vi "Codec_CMD_0_Will.vi"(8 "error in (no error)":errorcluster, 10 "CMD":u32, 11 "SecureMqttCodec in":refnum<class "SecureMqttCodec.lvclass">) -> (0 "error out":errorcluster, 2 "<JSON>":string, 3 "SecureMqttCodec out":refnum<class "SecureMqttCodec.lvclass">)   [LabVIEW 2020, in "SecureMqttCodec.lvclass"]
uses:
  SecureMqttCodec.lvclass
  SecureMqttCodec.lvclass/SecureMqttCodec.ctl
  <vilib>/LabVIEW Open Source Project/Epoch Date & Time/epoch.UNIX/Epoch.UNIX.lvclass
  C:/Program Files/National Instruments/LabVIEW 2020/vi.lib/LabVIEW Open Source Project/Epoch Date & Time/epoch/Epoch.lvclass
  <vilib>/addons/JSON API/JSON Scalar/JSON Scalar.lvclass
  C:/Program Files/National Instruments/LabVIEW 2020/vi.lib/addons/JSON API/JSON Value/JSON Value.lvclass
  <vilib>/LabVIEW Open Source Project/Epoch Date & Time/Get Epoch Time.vi
  <vilib>/addons/JSON API/JSON Scalar/Set I64.vi
  <vilib>/addons/JSON API/JSON Scalar/Set U32.vi
  <vilib>/addons/JSON API/JSON Scalar/Set String.vi
  <vilib>/addons/JSON API/JSON Value/Get as JSON string (pretty).vi
  <vilib>/addons/JSON API/JSON Value/JSON Value.lvclass
  <vilib>/addons/JSON API/Get Polymorphic/JSON GetSet.lvlib
panel:
  # "Command:\n0 -- Reg Client\n65535 -- Reg Will"
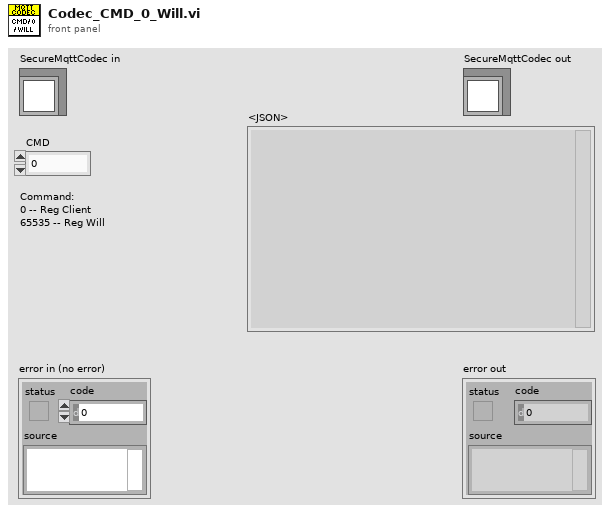
[diagram p1: front panel]
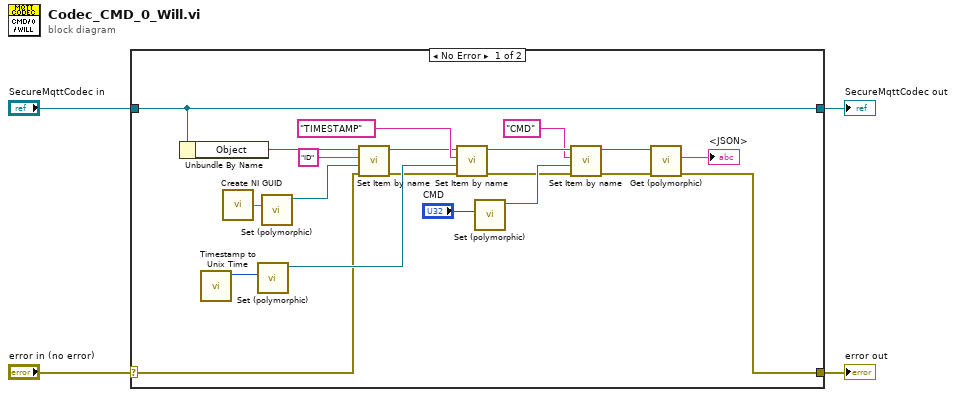
[diagram p0: block diagram]
diagram:
  n1 = case shown="No Error" "error in (no error)" {
    selector: "error in (no error)" -> [w9 w26]
    tunnel: [w6 w26] -> w3
    tunnel: [w24 w25] -> w1
    tunnel: "SecureMqttCodec in" -> [w24 w25]
    frame No Error {
      n2 = Unbundle By Name(w24) -> ("Object"=w23:refnum<class "JSON Value.lvclass">)
      n3 = call <vilib>:"Timestamp to Unix Time.vi"() -> ("Unix Time (s)"=w19:i64)  [unwired: 10 in, 1 out]
      n4 = call <vilib>:"Create NI GUID.vi"() -> ("NI GUID"=w21:string)
      n5 = call-poly <vilib>:"Set (polymorphic).vi"("Numeric"=w19) -> ("JSON Scalar out"=w18:refnum<class "JSON Scalar.lvclass">)  [unwired: 9 in, 1 out]
      n6 = call-poly <vilib>:"Set (polymorphic).vi"("String"=w21) -> ("JSON Scalar out"=w20:refnum<class "JSON Scalar.lvclass">)  [unwired: 9 in, 1 out]
      n7 = call-dynamic "Set Item by name.vi"("error in (no error)"=w9, "Value"=w20, "name"="ID", "JSON Value In"=w23) -> ("error out"=w15:errorcluster, "JSON Value Out"=w16:refnum<class "JSON Value.lvclass">)  [unwired: 5 in, 1 out]
      n8 = call-dynamic "Set Item by name.vi"("error in (no error)"=w15, "Value"=w18, "name"="TIMESTAMP", "JSON Value In"=w16) -> ("error out"=w10:errorcluster, "JSON Value Out"=w14:refnum<class "JSON Value.lvclass">)  [unwired: 5 in, 1 out]
      n9 = call-poly <vilib>:"Set (polymorphic).vi"("Numeric"="CMD") -> ("JSON Scalar out"=w12:refnum<class "JSON Scalar.lvclass">)  [unwired: 9 in, 1 out]
      n10 = call-dynamic "Set Item by name.vi"("error in (no error)"=w10, "Value"=w12, "name"="CMD", "JSON Value In"=w14) -> ("error out"=w7:errorcluster, "JSON Value Out"=w8:refnum<class "JSON Value.lvclass">)  [unwired: 5 in, 1 out]
      n11 = call-poly <vilib>:"Get (polymorphic).vi"("error in (no error)"=w7, "JSON Value in"=w8) -> ("error out"=w6:errorcluster, "<JSON>"=→"<JSON>":string)  [unwired: 8 in]
    }
    frame Error {
    }
  }
  "error out" <- w3
  "SecureMqttCodec out" <- w1
